vi "Self Execution.vi"(8 "error in (no error)":errorcluster, 9 "Task in":refnum<class "Task.lvclass">, 10 "Message In":refnum<class "Message.lvclass">, 11 "Actor In":refnum<class "System Actor.lvclass">) -> (0 "error out":errorcluster, 1 "Task out":refnum<class "Task.lvclass">, 2 "Message Out":refnum<class "Message.lvclass">, 3 "Actor Out":refnum<class "System Actor.lvclass">, 6 "Any Data":variant)   [LabVIEW 2019, in "Task.lvclass"]
uses:
  Task.lvclass
  Actor/System Actor/System Actor.lvclass
  Message/Message.lvclass
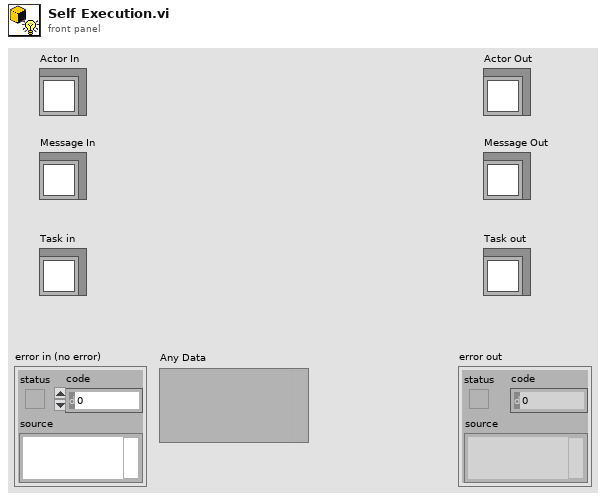
[diagram p1: front panel]
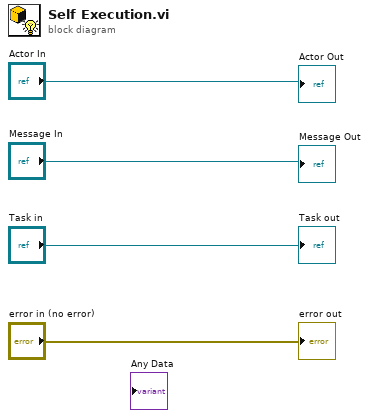
[diagram p0: block diagram]
diagram:
  "error out" <- "error in (no error)"
  "Task out" <- "Task in"
  "Actor Out" <- "Actor In"
  "Message Out" <- "Message In"
